vi "PCO_GetOffsetMode.vi"(8 "error in (no error)":errorcluster {"code" format="%x"}, 11 "ph":u64) -> (0 "error out":errorcluster {"code" format="%x"}, 1 "wOffsetRegulation":u16(ring) items=["AUTO", "OFF"], 2 "ErrorMessage":i32 format="%x", 3 "ph out":u64)   [LabVIEW 2019, in "SDK.lvlib" / "ImageSensor.lvlib"]
doc: "<b>Description:</b>\nThis function returns the current mode for the offset regulation with reference pixels (see respective camera manual for further explanations).\n\n<b>Supported camera type:</b>\npco.pixelfly usb, pco.ultraviolet, pco.1300, pco.1400\n\n<b>Descriptor dependency:</b>\nwOffsetRegulationDESC"
uses:
  ImageSensor.lvlib
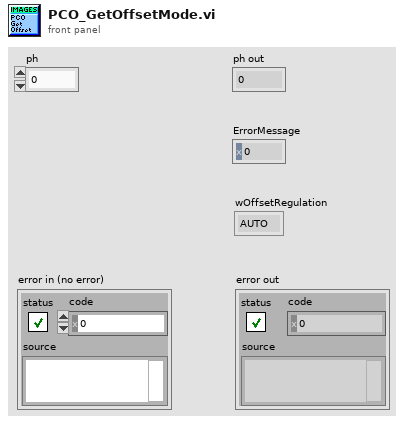
[diagram p1: front panel]
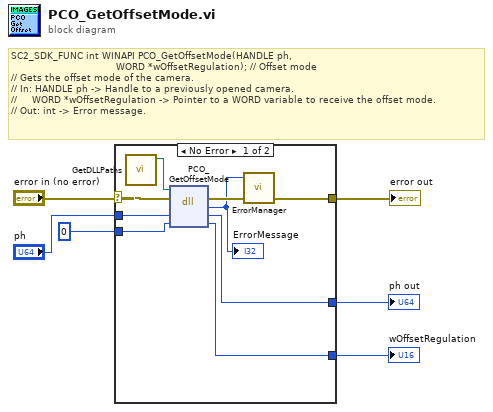
[diagram p0: block diagram]
diagram:
  # "SC2_SDK_FUNC int WINAPI PCO_GetOffsetMode(HANDLE ph,\n                                   WORD *wOffsetRegulation); // Offset mode\n// Gets the offset mode of the camera.\n// In: HANDLE ph -> Handle to a previously opened camera.\n//     WORD *wOffsetRegulation -> Pointer to a WORD variable to receive the offset mode.\n// Out: int -> Error message."
  n1 = case shown="No Error" "error in (no error)" {
    selector: "error in (no error)" -> [w9 w18]
    tunnel: "ph" -> [w15 w17]
    tunnel: [w14 w17] -> w5
    tunnel: u16 0 ("wOffsetRegulation") -> [w13 w16]
    tunnel: [w12 w16] -> w3
    tunnel: [w10 w18] -> w2
    frame No Error {
      n2 = call "GetDLLPaths.vi"() -> ("SC2_Cam_Path"=w7:path)  [unwired: 8 in, 3 out]
      n3 = dll-call lib="?" fn="PCO_GetOffsetMode"(path in=w7, error in=w9, "ph"=w15, "wOffsetRegulation"=w13) -> (error out=w11:errorcluster, "return type"=w8:i32, "ph"=w14:u64, "wOffsetRegulation"=w12:u16)  [unwired: 1 in, 1 out]
      "ErrorMessage" <- w8
      n4 = call "ErrorManager.vi"("error in (no error)"=w11, "error code"=w8) -> ("error out"=w10:errorcluster)  [unwired: 2 in, 1 out]
    }
    frame Error {
    }
  }
  "ph out" <- w5
  "wOffsetRegulation" <- w3
  "error out" <- w2
